vi "Voltage (non-regeneration) - Continuous Output.vi"() -> ()   [LabVIEW 2020]
uses:
  <vilib>/Utility/error.llb/DialogType.ctl
  <vilib>/DAQmx/write.llb/DAQmx Write (Analog 1D Wfm NChan NSamp).vi
  <vilib>/DAQmx/create/channels.llb/DAQmx Create Channel (AO-Voltage-Basic).vi
  <vilib>/DAQmx/configure/timing.llb/DAQmx Timing (Sample Clock).vi
  <vilib>/DAQmx/configure/trigger.llb/DAQmx Start Trigger (Digital Edge).vi
  <vilib>/DAQmx/configure/trigger.llb/DAQmx Start Trigger (Time).vi
  <vilib>/DAQmx/configure/trigger.llb/DAQmx Start Trigger (Analog Edge).vi
  <vilib>/DAQmx/miscellaneous.llb/DAQmx Fill In Error Info.vi
  <resource>/objmgr/daqmx.rc
  <vilib>/measure/NI_MABase.lvlib
panel:
  in  "Trigger Type":T1(tab)
  in  "Digital Start Trigger Edge":i32(ring)=10280 caption="Edge" items=["Rising"=10280, "Falling"=10171]
  in  "Digital Start Trigger Source":tag="/Dev1/PFI0" caption="Source"
  in  "Digital Pause Trigger Pause When":i32(ring)=10192 caption="Pause When" items=["High"=10192, "Low"=10214]
  in  "Digital Pause Trigger Source":tag="/Dev1/PFI0" caption="Source"
  in  "Analog Start Trigger Level":dbl caption="Level" format="%0.2f"
  in  "Analog Start Trigger Hysteresis":dbl caption="Hysteresis" format="%.2f"
  in  "Analog Start Trigger Slope":i32(ring)=10280 caption="Slope" items=["Rising"=10280, "Falling"=10171]
  in  "Analog Start Trigger Source":string="APFI0" caption="Source"
  in  "Analog Pause Trigger Source":string="APFI0" caption="Source"
  in  "Analog Pause Trigger Pause When":i32(ring)=10093 caption="Pause When" items=["Above Level"=10093, "Below Level"=10107]
  in  "Analog Pause Trigger Level":dbl caption="Level" format="%.2f"
  in  "When":timestamp
  in  "Select Time\nManually":bool
  in  "Output Array":T2(array[cluster])=[{"Waveform Type"=0, "Amplitude"=1.0, "Frequency"=17.0}] {"Frequency" format="%0.2p"; "Amplitude" format="%0.2p"; "Waveform Type" items=["Sine Wave", "Triangle Wave", "Square Wave", "Sawtooth Wave"]}
  in  "Number of Samples":i32=1000
  in  "Stop":bool
  out "Waveform Graph":waveform(dbl)[](graph)=[{"t0"=timestamp(0 s since 1904-01-01), "dt"=0.001, "Y"=[]}]
  in  "Sample Rate":dbl=1000.0
  in  "Sample Clock Source":tag="OnboardClock"
  in  "Max Voltage":dbl=5.0
  in  "Min Voltage":dbl=-5.0
  in  "Physical Channel(s)":tag="Dev1/ao0"
  out "Actual Sample Rate":dbl=1000.0 format="%0.2f"
  # "Channel Settings"
  # "Output"
  # "Timing and Buffer Settings"
  # "Waveform Settings"
  # "Trigger Settings"
  # "The number of elements in the waveform array\nmust equal the number of channels in the task."
  # "To enable triggers, select a tab above, and configure the settings.\n\nNot all hardware supports all trigger types. Refer to your device documentation for more information."
  # "This trigger type is not supported in output tasks. \n\nRefer to your device documentation for more information on which triggers are supported."
  # "This trigger type is not supported in output tasks. \n\nRefer to your device documentation for more information on which triggers are supported."
  # "If time is not manually set, task will begin after 10 seconds"
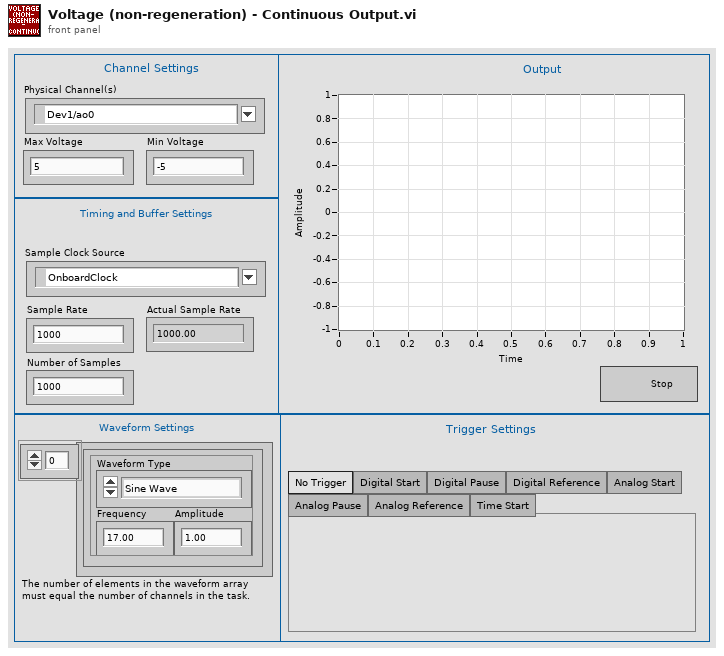
[diagram p1: front panel]
types:
  T1 = enum32{"No Trigger", "Digital Start", "Digital Pause", "Digital Reference", "Analog Start", "Analog Pause", "Analog Reference", "Time Start"}
  T2 = cluster{"Waveform Type":u16, "Amplitude":dbl, "Frequency":dbl}[]
  T3 = typedef "DialogType.ctl" = u16
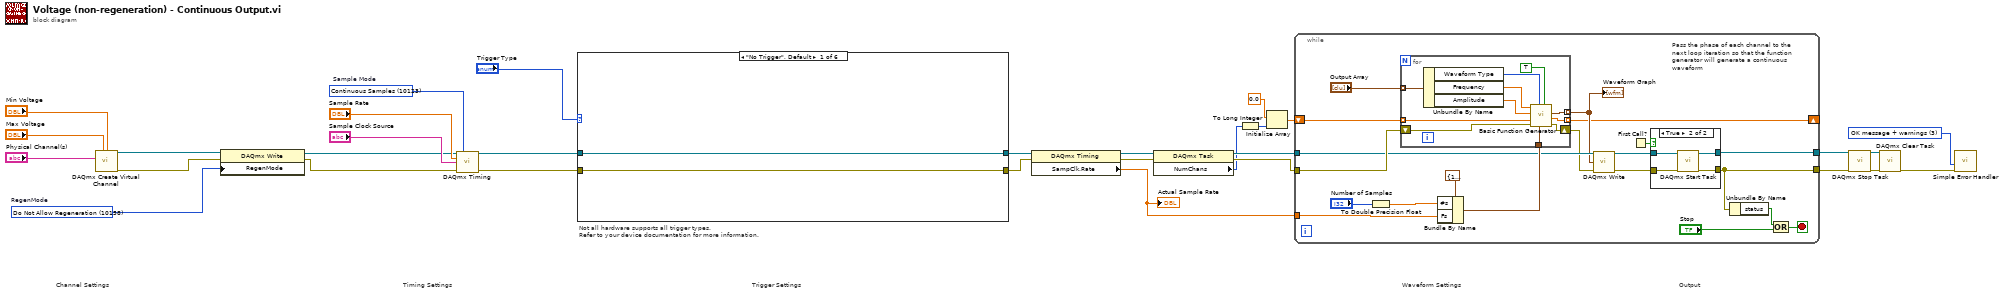
[diagram p0: block diagram]
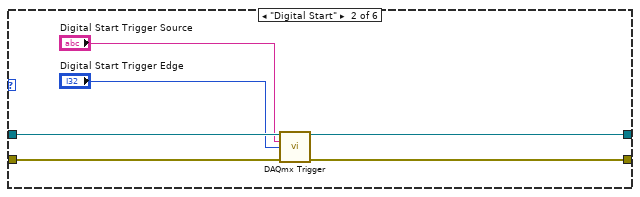
[diagram p2: hidden frame]
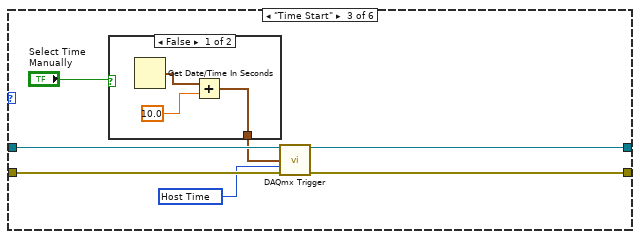
[diagram p3: hidden frame]
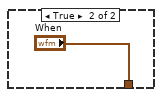
[diagram p4: hidden frame]
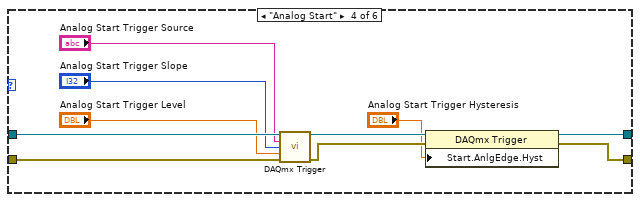
[diagram p5: hidden frame]
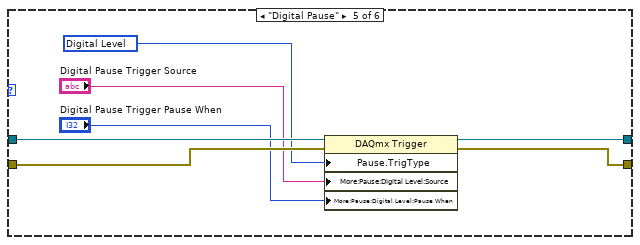
[diagram p6: hidden frame]
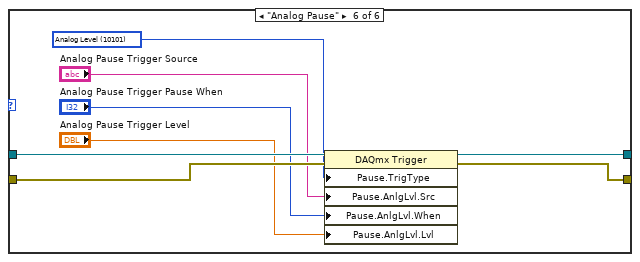
[diagram p7: hidden frame]
diagram:
  w14 = T3 3 items=["no dialog", "OK message", "continue or stop message", "OK message + warnings", "continue/stop + warnings"] ("type of dialog (OK msg:1)")
  w21 = 10158 items=["Allow Regeneration"=10097, "Do Not Allow Regeneration"=10158]  # RegenMode
  w31 = 10123 items=["Finite Samples"=10178, "Continuous Samples"=10123, "Hardware Timed Single Point"=12522]  # Sample Mode
  # "Trigger Settings"
  # "Not all hardware supports all trigger types.\nRefer to your device documentation for more information."
  # "Output"
  # "Waveform Settings"
  # "Timing Settings"
  # "Channel Settings"
  n1 = call-poly <vilib>:"DAQmx Create Virtual Channel.vi"("maximum value"="Max Voltage", "minimum value"="Min Voltage", "physical channels"="Physical Channel(s)") -> ("task out"=w23:refnum<k21>, "error out"=w22:errorcluster)  [unwired: 11 in]
  n2 = property class="DAQmx Write"(reference=w23, error in=w22, "RegenMode"=w21) -> (reference out=w19:refnum<k21>, error out=w20:errorcluster)
  n3 = call-poly <vilib>:"DAQmx Timing.vi"("task/channels in"=w19, "sample mode"=w31, "rate"="Sample Rate", "source"="Sample Clock Source", "error in"=w20) -> ("task out"=w3:refnum<k21>, "error out"=w4:errorcluster)  [unwired: 9 in]
  n4 = case shown="\"No Trigger\", Default" "Trigger Type" {
    tunnel: w3 -> [w33 w39 w46 w60 w67 w75]
    tunnel: w4 -> [w32 w38 w45 w59 w64 w72]
    tunnel: [w33 w37 w44 w57 w66 w74] -> w2
    tunnel: [w32 w36 w43 w56 w65 w73] -> w1
    frame "No Trigger", Default {
    }
    frame "Digital Start" {
      n5 = call-poly <vilib>:"DAQmx Trigger.vi"("task/channels in"=w39, "source"="Digital Start Trigger Source", "edge"="Digital Start Trigger Edge", "error in"=w38) -> ("task out"=w37:refnum<k21>, "error out"=w36:errorcluster)  [unwired: 10 in]
    }
    frame "Time Start" {
      w40 = 16126 items=["Host Time"=16126, "I/O Device Time"=16127] ("timescale")
      n6 = case shown="False" "Select Time\nManually" {
        tunnel: [w48 "When"] -> w41
        frame False {
          n7 = Get Date/Time In Seconds() -> (seconds since 1Jan1904=w49:timestamp)
          n8 = Add(x=w49, y=10.0) -> (x+y=w48:timestamp)
        }
        frame True {
        }
      }
      n9 = call-poly <vilib>:"DAQmx Trigger.vi"("task/channels in"=w46, "when"=w41, "timescale"=w40, "error in"=w45) -> ("task out"=w44:refnum<k21>, "error out"=w43:errorcluster)  [unwired: 10 in]
    }
    frame "Analog Start" {
      n10 = call-poly <vilib>:"DAQmx Trigger.vi"("task/channels in"=w60, "source"="Analog Start Trigger Source", "slope"="Analog Start Trigger Slope", "level"="Analog Start Trigger Level", "error in"=w59) -> ("task out"=w55:refnum<k21>, "error out"=w54:errorcluster)  [unwired: 9 in]
      n11 = property class="DAQmx Trigger"(reference=w55, error in=w54, "Start.AnlgEdge.Hyst"="Analog Start Trigger Hysteresis") -> (reference out=w57:refnum<k21>, error out=w56:errorcluster)
    }
    frame "Digital Pause" {
      w63 = 10152 items=["Analog Level"=10101, "Analog Window"=10103, "Digital Level"=10152, "Digital Pattern"=10398, "None"=10230] ("Pause.TrigType")
      n12 = property class="DAQmx Trigger"(reference=w67, error in=w64, "Pause.TrigType"=w63, "More:Pause:Digital Level:Source"="Digital Pause Trigger Source", "More:Pause:Digital Level:Pause When"="Digital Pause Trigger Pause When") -> (reference out=w66:refnum<k21>, error out=w65:errorcluster)
    }
    frame "Analog Pause" {
      w71 = 10101 items=["Analog Level"=10101, "Analog Window"=10103, "Digital Level"=10152, "Digital Pattern"=10398, "None"=10230] ("Pause.TrigType")
      n13 = property class="DAQmx Trigger"(reference=w75, error in=w72, "Pause.TrigType"=w71, "Pause.AnlgLvl.Src"="Analog Pause Trigger Source", "Pause.AnlgLvl.When"="Analog Pause Trigger Pause When", "Pause.AnlgLvl.Lvl"="Analog Pause Trigger Level") -> (reference out=w74:refnum<k21>, error out=w73:errorcluster)
    }
  }
  n14 = property class="DAQmx Timing"(reference=w2, error in=w1) -> (reference out=w9:refnum<k21>, error out=w8:errorcluster, "SampClk.Rate"=w24:dbl)
  "Actual Sample Rate" <- w24
  n15 = property class="DAQmx Task"(reference=w9, error in=w8) -> (reference out=w11:refnum<k21>, error out=w10:errorcluster, "NumChans"=w7:u32)
  n16 = To Long Integer(number=w7) -> (32bit integer=w6:i32)
  n17 = Initialize Array(0.0 ("element"), w6) -> (w12:dbl[])
  n18 = while {
    tunnel: w10 -> [w95]
    tunnel: w24 -> [w93]
    tunnel: w11 -> [w91]
    tunnel: [w82] -> w16
    tunnel: [w81] -> w15
    shift-right: [w77] -> _
    shift-left: w12 -> [w76]
    stop <- w79 stop-if-true
    # "Pass the phase of each channel to the next loop iteration so that the function generator will generate a continuous waveform"
    n19 = To Double Precision Float(number="Number of Samples") -> (double precision float=w85:dbl)
    n20 = Bundle By Name(cluster=cluster{"Fs":dbl, "#s":dbl} {"Fs"=1000.0, "#s"=1000.0} ("sampling info"), "#s"=w85, "Fs"=w93) -> (w92:cluster{"Fs":dbl, "#s":dbl})
    n21 = for {
      tunnel: w92 -> [w111]
      tunnel: "Output Array" -> [w109] mode=indexing
      tunnel: [w105] -> w86 mode=indexing
      tunnel: [w104] -> w77 mode=indexing
      tunnel: w76 -> [w102] mode=indexing
      shift-right: [w110] -> w88
      shift-left: w95 -> [w112]
      n22 = Unbundle By Name(w109) -> ("Waveform Type"=w108:u16, "Frequency"=w107:dbl, "Amplitude"=w106:dbl)
      n23 = call <vilib>:"Basic Function Generator.vi"("reset signal"=TRUE, "sampling info"=w111, "signal type"=w108, "error in (no error)"=w112, "phase"=w102, "amplitude"=w106, "frequency"=w107) -> ("error out"=w110:errorcluster, "phase out"=w104:dbl, "signal out"=w105:waveform(dbl))  [unwired: 2 in]
    }
    "Waveform Graph" <- w86
    n24 = call-poly <vilib>:"DAQmx Write.vi"("task/channels in"=w91, "data"=w86, "error in"=w88) -> ("task out"=w90:refnum<k21>, "error out"=w89:errorcluster)  [unwired: 10 in, 1 out]
    n25 = First Call?() -> (First Call?: T/F=w83:bool)
    n26 = case shown="True" w83 {
      tunnel: w90 -> [w96 w101]
      tunnel: w89 -> [w97 w100]
      tunnel: [w96 w99] -> w82
      tunnel: [w97 w98] -> w81
      frame False {
      }
      frame True {
        n27 = call <vilib>:"DAQmx Start Task.vi"("task/channels in"=w101, "error in"=w100) -> ("task out"=w99:refnum<k21>, "error out"=w98:errorcluster)  [unwired: 12 in]
      }
    }
    n28 = Unbundle By Name(w81) -> ("status"=w78:bool)
    n29 = Or(x=w78, y="Stop") -> (x .or. y?=w79:bool)
  }
  n30 = call <vilib>:"DAQmx Stop Task.vi"("task/channels in"=w16, "error in"=w15) -> ("task out"=w18:refnum<k21>, "error out"=w17:errorcluster)  [unwired: 12 in]
  n31 = call <vilib>:"DAQmx Clear Task.vi"("task in"=w18, "error in"=w17) -> ("error out"=w30:errorcluster)  [unwired: 13 in]
  n32 = call <vilib>:"Simple Error Handler.vi"("type of dialog (OK msg:1)"=w14, "error in (no error)"=w30) -> ()  [unwired: 3 in, 5 out]
